vi "Un(Re)doTblChng.vi"(5 "Undo/Redo":enum16{"Undo", "Redo"}(ring), 6 "ModeCol Index":i32=2, 7 "Layout Ref":refnum<vi>, 8 "error in (no error)":errorcluster, 9 "Table CtlRef In":refnum<vi>, 10 "Col Array in":refnum<class "Column.lvclass">[](array[class]), 11 "Table History ref":refnum<vi>) -> (0 "error out":errorcluster)   [LabVIEW 2013]
doc: "Depending on Undo/Redo enum:\n undo: Swap current Table with older History + increment internal pointer;\n redo: decrement internal pointer + swap current Table with newer History.\n\nThis VI is read-only w.r.t Column Array."
uses:
  TypeDefs/TableHistory.ctl
  TypeDefs/TableArray.ctl
  ColumnVIs/Column/Column.lvclass
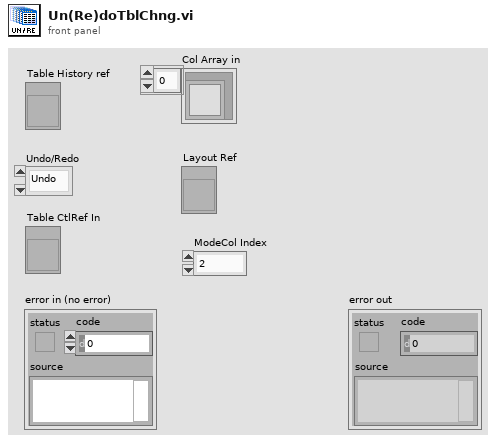
[diagram p1: front panel]
types:
  T1 = typedef "TableHistory.ctl" = cluster{"OldTable Array":T2, "Undo pointer":i32}
  T2 = typedef "TableArray.ctl" = cluster{"OldTable":string[][]}[]
  T3 = typedef "LVRowAndColumnTypeDef.ctl" = cluster{"Row":i32, "Column":i32}
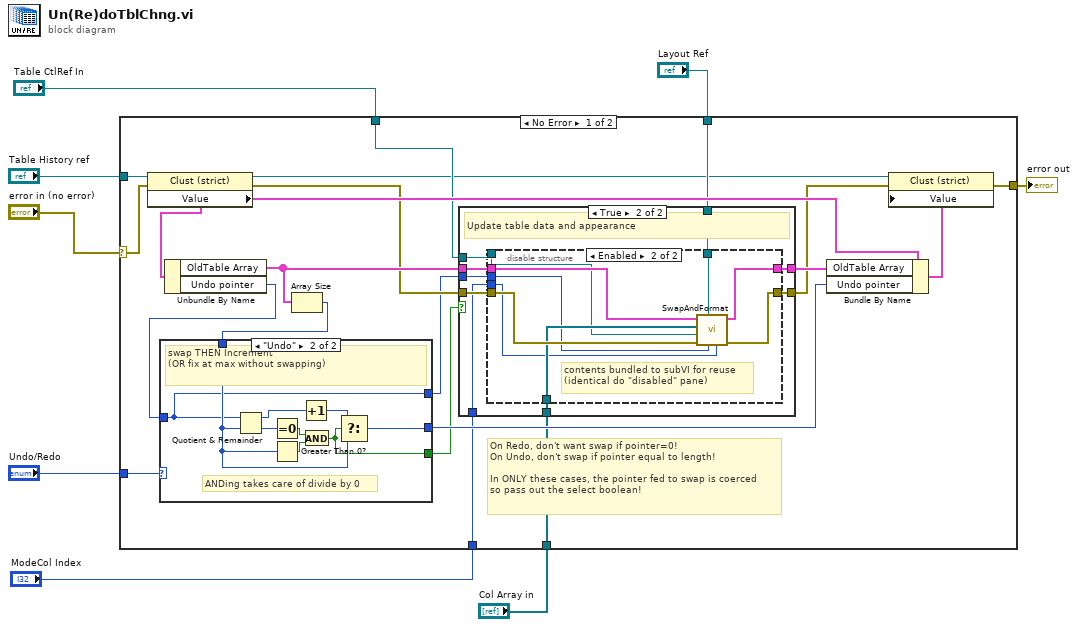
[diagram p0: block diagram]
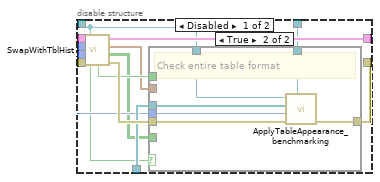
[diagram p3: hidden frame]
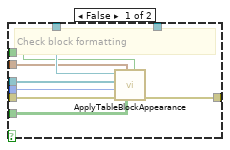
[diagram p4: hidden frame]
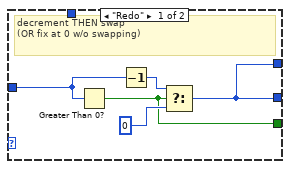
[diagram p5: hidden frame]
diagram:
  n1 = case shown="No Error" "error in (no error)" {
    selector: "error in (no error)" -> [w17 w91]
    tunnel: "Undo/Redo" -> [w28 _]
    tunnel: "Table History ref" -> [w27 _]
    tunnel: [w12 w91] -> w6
    tunnel: "Table CtlRef In" -> [w14 _]
    tunnel: "Col Array in" -> [w10 _]
    tunnel: "Layout Ref" -> [w11 _]
    tunnel: "ModeCol Index" -> [w13 _]
    frame No Error {
      # "On Redo, don't want swap if pointer=0!\nOn Undo, don't swap if pointer equal to length!\n\nIn ONLY these cases, the pointer fed to swap is coerced\nso pass out the select boolean!"
      n2 = property class="Clust (strict)"(reference=w27, error in=w17) -> (reference out=w9:refnum<vi>, error out=w20:errorcluster, "Value"=w25:T1)
      n3 = Unbundle By Name(w25) -> ("OldTable Array"=w22:T2, "Undo pointer"=w16:i32)
      n4 = Array Size(array=w22) -> (size(s)=w26:i32)
      n5 = case shown="\"Undo\"" w28 {
        tunnel: w16 -> [w80 w83]
        tunnel: [w78 w87] -> w23
        tunnel: [w78 w83] -> w18
        tunnel: w26 -> [_ w86]
        tunnel: [w77 w82] -> w15
        frame "Redo" {
          # "decrement THEN swap\n(OR fix at 0 w/o swapping)"
          n6 = Greater Than 0?(x=w80) -> (x > 0?=w77:bool)
          n7 = Decrement(x=w80) -> (x-1=w79:i32)
          n8 = Select(t=w79, s=w77, f=0) -> (s? t:f=w78:i32)
        }
        frame "Undo" {
          # "ANDing takes care of divide by 0"
          # "swap THEN Increment\n(OR fix at max without swapping)"
          n9 = Quotient & Remainder(x=w83, y=w86) -> (x-y*floor(x/y)=w89:i32, floor(x/y)=w90:i32)
          n10 = Equal To 0?(x=w90) -> (x = 0?=w85:bool)
          n11 = Greater Than 0?(x=w86) -> (x > 0?=w84:bool)
          n12 = Increment(x=w89) -> (x+1=w88:i32)
          n13 = And(x=w85, y=w84) -> (x .and. y?=w82:bool)
          n14 = Select(t=w88, s=w82, f=w86) -> (s? t:f=w87:i32)
        }
      }
      n15 = case shown="True" w15 {
        tunnel: w22 -> [w30 w39]
        tunnel: [w30 w38] -> w21
        tunnel: w20 -> [w29 w37]
        tunnel: [w29 w35] -> w19
        tunnel: w18 -> [_ w36]
        tunnel: w14 -> [_ w34]
        tunnel: w13 -> [_ w31]
        tunnel: w11 -> [_ w33]
        tunnel: w10 -> [_ w32]
        frame False {
          # "at oldest/newest change: do nothing!"
        }
        frame True {
          # "Update table data and appearance"
          n16 = disable-structure shown="Enabled" {
            disable-tunnel: w39 -> [w53 w73]
            disable-tunnel: [w52 w72] -> w38
            disable-tunnel: w37 -> [w51 w75]
            disable-tunnel: w36 -> [w50 w69]
            disable-tunnel: [w48 w76] -> w35
            disable-tunnel: w34 -> [w47 w70]
            disable-tunnel: w33 -> [w46 w71]
            disable-tunnel: w32 -> [w45 w74]
            disable-tunnel: w31 -> [w44 w68]
            frame Disabled {
              n17 = call "SwapWithTblHist.vi"("Table CtlRef In"=w47, "error in (no error)"=w51, "Mode Index"=w44, "Undo pointer"=w50, "OldTable Array in"=w53) -> ("error out"=w49:errorcluster, "changed? subarray"=w41:bool[][], "Change start"=w40:T3, "OldTable Array out"=w52:T2, "Mode change?"=w42:bool, "Size mismatch?"=w43:bool)  [unwired: 1 in]
              n18 = case shown="True" w43 {
                tunnel: w49 -> [w61 w67]
                tunnel: [w60 w66] -> w48
                tunnel: w47 -> [w59 w65]
                tunnel: w46 -> [_ w64]
                tunnel: w45 -> [w58 w63]
                tunnel: w44 -> [w57 w62]
                tunnel: w42 -> [w56 _]
                tunnel: w41 -> [w55 _]
                tunnel: w40 -> [w54 _]
                frame False {
                  # "Check block formatting"
                  n19 = call "ApplyTableBlockAppearance.vi"("Check Mode?"=w56, "changed? subarray"=w55, "Change start"=w54, "error in (no error)"=w61, "Mode Index"=w57, "Col Array in"=w58, "Table Ref in"=w59) -> ("error out"=w60:errorcluster)  [unwired: 4 in]
                }
                frame True {
                  # "Check entire table format"
                  n20 = call "ApplyTableAppearance_benchmarking.vi"("Layout Ring Ref"=w64, "error in (no error)"=w67, "Mode Index"=w62, "Col Array in"=w63, "Table Ref in"=w65) -> ("error out"=w66:errorcluster)  [unwired: 5 in, 1 out]
                }
              }
            }
            frame Enabled {
              # "contents bundled to subVI for reuse\n(identical do \"disabled\" pane)"
              n21 = call "SwapAndFormat.vi"("Mode Index"=w68, "Undo pointer"=w69, "Layout Ref"=w71, "error in (no error)"=w75, "Table CtlRef In"=w70, "Col Array in"=w74, "OldTable Array in"=w73) -> ("error out"=w76:errorcluster, "OldTable Array out"=w72:T2)  [unwired: 3 in]
            }
          }
        }
      }
      n22 = Bundle By Name(cluster=w25, "OldTable Array"=w21, "Undo pointer"=w23) -> (w24:T1)
      n23 = property class="Clust (strict)"(reference=w9, error in=w19, "Value"=w24) -> (error out=w12:errorcluster)  [unwired: 1 out]
    }
    frame Error {
    }
  }
  "error out" <- w6
